vi "Set Running.vi"(8 "error in (no error)":errorcluster, 10 "Running":bool, 11 "Common Measurements Interface in":refnum<class "Common Measurements Interface.lvclass">) -> (0 "error out":errorcluster, 3 "Common Measurements Interface out":refnum<class "Common Measurements Interface.lvclass">)   [LabVIEW 2015, in "Common Measurements Interface.lvclass"]
uses:
  Common Measurements Interface.lvclass
  Common Measurements Interface.lvclass/Common Measurements Interface.ctl
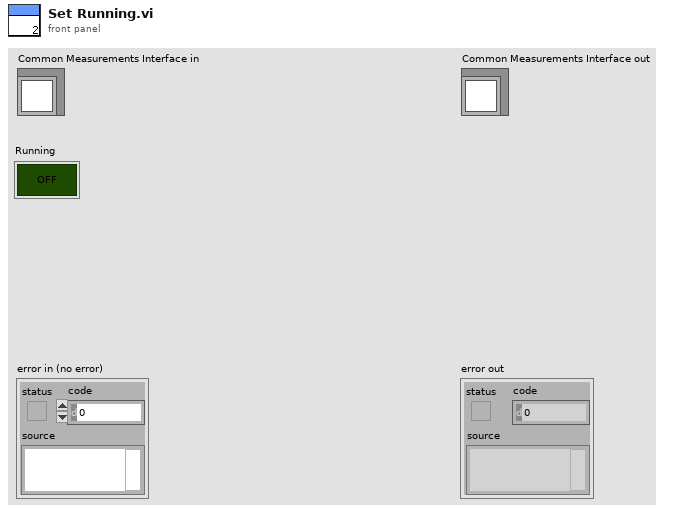
[diagram p1: front panel]
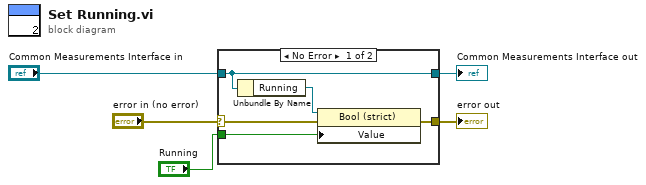
[diagram p0: block diagram]
diagram:
  n1 = case shown="No Error" "error in (no error)" {
    selector: "error in (no error)" -> [w7 w12]
    tunnel: [w6 w12] -> w4
    tunnel: [w10 w11] -> w2
    tunnel: "Common Measurements Interface in" -> [w10 w11]
    tunnel: "Running" -> [w8 _]
    frame No Error {
      n2 = Unbundle By Name(w10) -> ("Running"=w9:refnum<vi>)
      n3 = property class="Bool (strict)"(reference=w9, error in=w7, "Value"=w8) -> (error out=w6:errorcluster)  [unwired: 1 out]
    }
    frame Error {
    }
  }
  "error out" <- w4
  "Common Measurements Interface out" <- w2
